vi "create Receipt.vi"(6 "Date":timestamp, 7 "Account":string, 8 "error in (no error)":errorcluster, 9 "Store":T1, 10 "Amount":dbl, 11 "Receipt in":refnum<class "Receipt.lvclass">) -> (0 "error out":errorcluster, 3 "Receipt out":refnum<class "Receipt.lvclass">)   [LabVIEW 2020, in "Receipt.lvclass"]
uses:
  Receipt.lvclass
  Receipt.lvclass/Receipt.ctl
  AReceipt/Store STYP.ctl
  AReceipt/AReceipt.lvclass
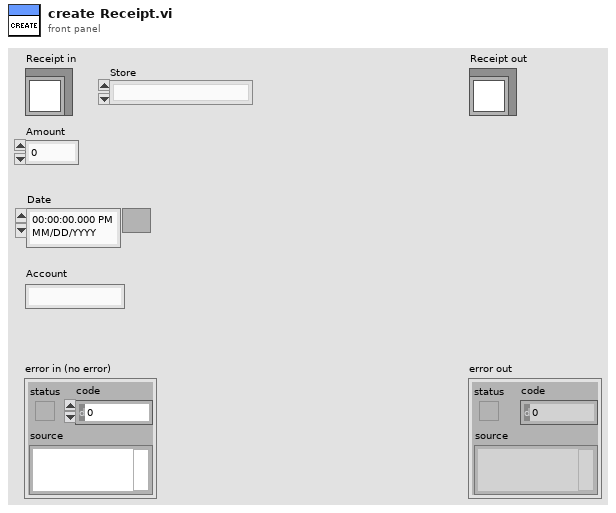
[diagram p1: front panel]
types:
  T1 = typedef "AReceipt.lvclass/Store STYP.ctl" = enum16{""}
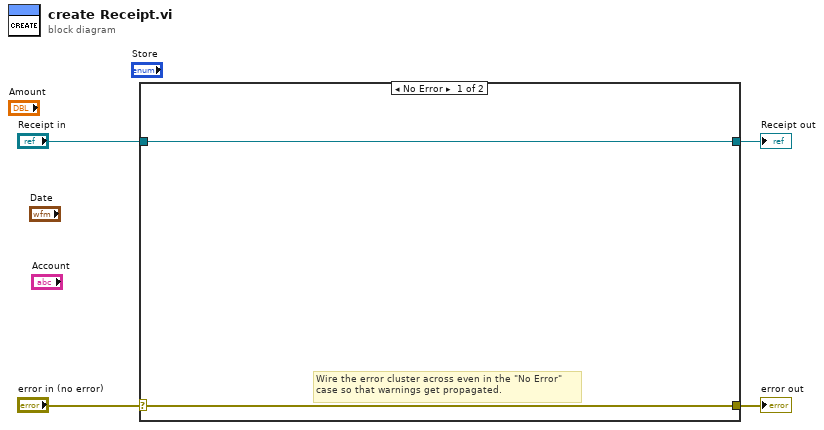
[diagram p0: block diagram]
diagram:
  n1 = case shown="No Error" "error in (no error)" {
    selector: "error in (no error)" -> [w5 w8]
    tunnel: [w5 w8] -> w3
    tunnel: [w6 w7] -> w1
    tunnel: "Receipt in" -> [w6 w7]
    frame No Error {
      # "Wire the error cluster across even in the \"No Error\"\ncase so that warnings get propagated."
    }
    frame Error {
    }
  }
  "error out" <- w3
  "Receipt out" <- w1
